vi "BME_DG_InitializeMultipleBus.vi"(6 "BusNr":i32, 7 "error in (no error)":errorcluster, 8 "Slot Number":i32, 9 "DG_Product":i32, 10 "DG_Number":i32) -> (0 "error out":errorcluster)   [LabVIEW 2009, in "POLARIS BME DG.lvlib"]
uses:
  POLARIS BME DG.lvlib
  BME DLL/DelayGenerator.dll
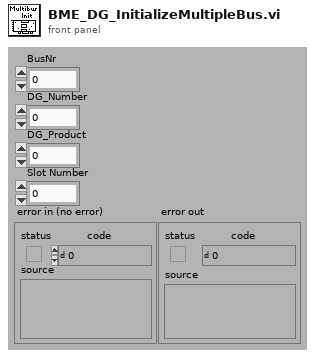
[diagram p1: front panel]
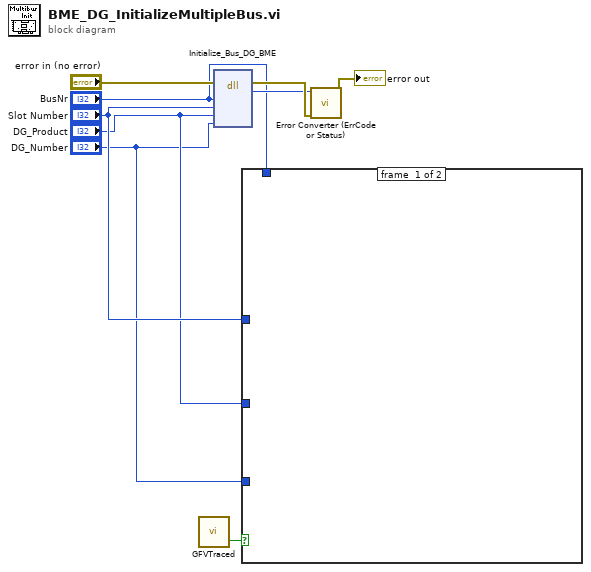
[diagram p0: block diagram]
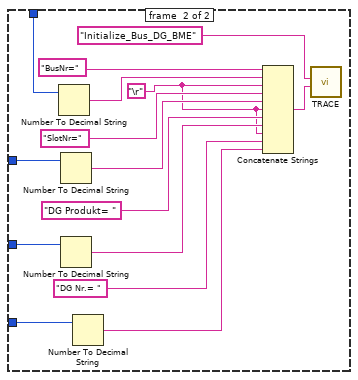
[diagram p2: hidden frame]
diagram:
  n1 = call "GFVTraced.vi"() -> ("traced?"=w5:bool)  [unwired: 2 in]
  n2 = dll-call lib="D:/CS Framework/LVSCC/LV2009/GPL/Projects/cs-framework/CSClass/CSPOLARIS/POLARIS BME DG/BME DLL/DelayGenerator.dll" fn="Initialize_Bus_DG_BME"(error in="error in (no error)", "BusNr"="BusNr", "SlotNr"="Slot Number", "ProductID"="DG_Product", "DG_Number"="DG_Number") -> (error out=w8:errorcluster, "return type"=w6:i32)  [unwired: 6 in, 1 out]
  n3 = case shown="True" w5 {
    tunnel: "BusNr" -> [_ w22]
    tunnel: "Slot Number" -> [_ w18]
    tunnel: "DG_Product" -> [_ w17]
    tunnel: "DG_Number" -> [_ w11]
    frame #0 {
    }
    frame #1 {
      w14 = "\r"
      n4 = Number To Decimal String(number=w22) -> (decimal integer string=w21:string)  [unwired: 1 in]
      n5 = Number To Decimal String(number=w18) -> (decimal integer string=w19:string)  [unwired: 1 in]
      n6 = Number To Decimal String(number=w17) -> (decimal integer string=w15:string)  [unwired: 1 in]
      n7 = Number To Decimal String(number=w11) -> (decimal integer string=w12:string)  [unwired: 1 in]
      n8 = Concatenate Strings("BusNr=", w21, w14, "SlotNr=", w19, w14, "DG Produkt= ", w15, w14, "DG Nr.= ", w12) -> (w10:string)
      n9 = call "TRACE.vi"("Parameter String"=w10, "Function"="Initialize_Bus_DG_BME") -> ()  [unwired: 10 in]
    }
  }
  n10 = call "Error Converter (ErrCode or Status).vi"("error in (no error)"=w8, "error code"=w6) -> ("error out"=→"error out":errorcluster)  [unwired: 9 in]
